vi "Configure DUT Loss Compensation.vi"(0 "VISA resource name":refnum<visa-resource-name>, 1 "Compensation Type (0: After)":u16(ring) items=["After", "Before"], 5 "Compensation Method (0: Off)":u16(ring) items=["Off", "Table", "Fixed"], 7 "DUT Loss Compensation Fixed Value (0 dB)":dbl, 9 "DUT Loss Compensation Table (Frequency/Amplitude)":dbl[][](array[numeric]) format="%^#_6g", 11 "error in (no error)":errorcluster) -> (4 "VISA resource name out":refnum<visa-resource-name>, 15 "error out":errorcluster)   [LabVIEW 2014, in "Agilent ESA PSA Series.lvlib"]
doc: "Enables and configures or disables the Dut Loss compensation mode of the Noise Figure personality.\n\n<B>Note:</B> \n\nThis VI is only valid in Noise Figure personality. Use <B>Switch Personality</B> VI to switch to Noise Figure before calling this VI."
uses:
  Agilent ESA PSA Series.lvlib
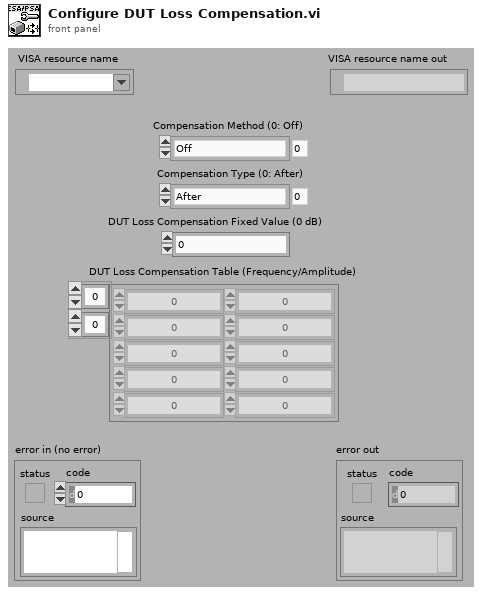
[diagram p1: front panel]
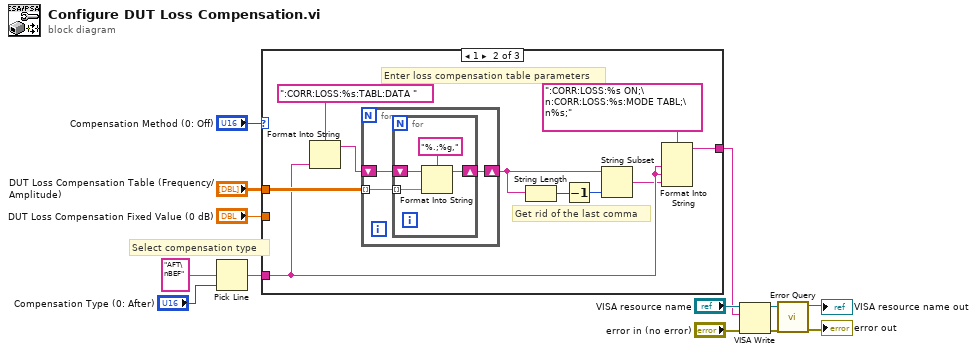
[diagram p0: block diagram]
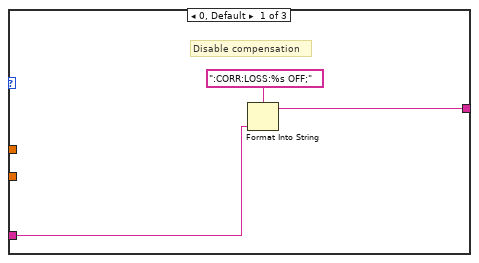
[diagram p2: hidden frame]
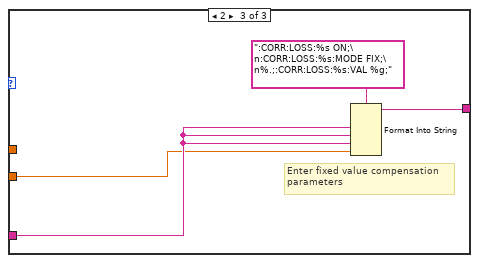
[diagram p3: hidden frame]
diagram:
  # "Select compensation type"
  n1 = Pick Line(multi-line string="AFT\nBEF", line index="Compensation Type (0: After)") -> (output string=w1:string)  [unwired: 1 in]
  n2 = case shown="1" "Compensation Method (0: Off)" {
    tunnel: [w14 w23 w37] -> w7
    tunnel: "DUT Loss Compensation Table (Frequency/Amplitude)" -> [_ w21 _]
    tunnel: "DUT Loss Compensation Fixed Value (0 dB)" -> [_ _ w34]
    tunnel: w1 -> [w15 w18 w35]
    frame 0, Default {
      # "Disable compensation"
      n3 = Format Into String(format string=":CORR:LOSS:%s OFF;", w15) -> (resulting string=w14:string)  [unwired: 2 in, 1 out]
    }
    frame 1 {
      # "Enter loss compensation table parameters"
      # "Get rid of the last comma"
      n4 = Format Into String(format string=":CORR:LOSS:%s:TABL:DATA ", w18) -> (resulting string=w19:string)  [unwired: 2 in, 1 out]
      n5 = for {
        tunnel: w21 -> [w29] mode=indexing
        shift-right: [w27] -> w24
        shift-left: w19 -> [w28]
        n6 = for {
          tunnel: w29 -> [w33] mode=indexing
          shift-right: [w31] -> w27
          shift-left: w28 -> [w32]
          n7 = Format Into String(format string="%.;%g,", initial string=w32, w33) -> (resulting string=w31:string)  [unwired: 1 in, 1 out]
        }
      }
      n8 = String Length(string=w24) -> (length=w25:i32)
      n9 = Decrement(x=w25) -> (x-1=w26:i32)
      n10 = String Subset(string=w24, length (rest)=w26) -> (substring=w17:string)  [unwired: 1 in]
      n11 = Format Into String(format string=":CORR:LOSS:%s ON;\n:CORR:LOSS:%s:MODE TABL;\n%s;", w18, w18, w17) -> (resulting string=w23:string)  [unwired: 2 in, 1 out]
    }
    frame 2 {
      # "Enter fixed value compensation\nparameters"
      n12 = Format Into String(format string=":CORR:LOSS:%s ON;\n:CORR:LOSS:%s:MODE FIX;\n%.;:CORR:LOSS:%s:VAL %g;" ("initial string"), w35, w35, w35, w34) -> (resulting string=w37:string)  [unwired: 2 in, 1 out]
    }
  }
  n13 = VISA Write(VISA resource name="VISA resource name", write buffer=w7, error in (no error)="error in (no error)") -> (VISA resource name out=w8:refnum<visa-resource-name>, error out=w10:errorcluster)  [unwired: 1 out]
  n14 = call "Error Query.vi"("error in (no error)"=w10, "VISA resource name"=w8) -> ("error out"=→"error out":errorcluster, "VISA resource name out"=→"VISA resource name out":refnum<visa-resource-name>)  [unwired: 6 in, 2 out]
